vi "xy_ref_lpf.vi"(6 "enable":bool, 7 "lpf-Order":i32=2, 8 "Den":sgl[](array[numeric])=[0.982758, -1.98194, 1.0, 0.0, 0.0, 0.0, 0.0, 0.0, 0.0], 9 "Num":sgl[](array[numeric])=[-0.00254, 0.000408, 0.00295, 0.0, 0.0, 0.0, 0.0, 0.0, 0.0], 11 "xy_ref":fxp<+/-,16,5>[](array[numeric])=[0.0, 0.0]) -> (3 "xy_ref_filt":fxp<+/-,16,5>[](array[numeric]))   [LabVIEW 2017]
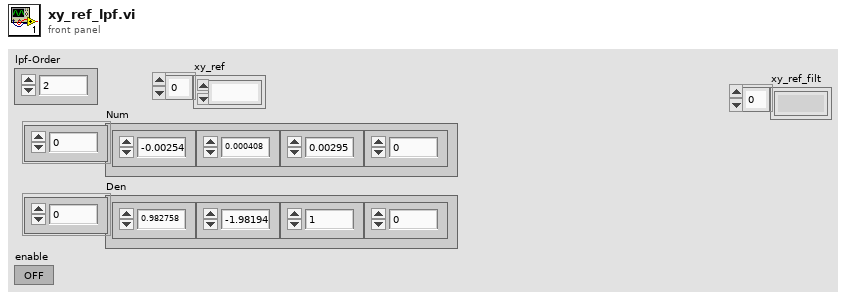
[diagram p1: front panel]
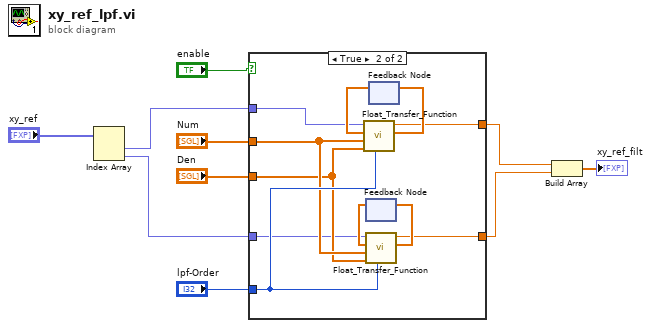
[diagram p0: block diagram]
diagram:
  n1 = Index Array(array="xy_ref") -> (element #1=w5:fxp<+/-,16,5>, element #2=w4:fxp<+/-,16,5>)  [unwired: 2 in]
  n2 = case shown="True" "enable" {
    tunnel: "lpf-Order" -> [_ w23]
    tunnel: "Num" -> [_ w22]
    tunnel: "Den" -> [_ w21]
    tunnel: [w12 w16] -> w2
    tunnel: [w11 w15] -> w1
    tunnel: w5 -> [w12 w14]
    tunnel: w4 -> [w11 w13]
    frame False {
    }
    frame True {
      n3 = feedback #1() -> (w19:sgl[])  [unwired: 1 in]
      n4 = call "Float_Transfer_Function.vi"("TF Order"=w23, "Den"=w21, "Num"=w22, "State In"=w19, "Input"=w13) -> ("State Out"=w20:sgl[], "Output"=w15:sgl)  [unwired: 4 in]
      n5 = feedback-in #1(w20) -> ()
      n6 = feedback #2() -> (w17:sgl[])  [unwired: 1 in]
      n7 = call "Float_Transfer_Function.vi"("TF Order"=w23, "Den"=w21, "Num"=w22, "State In"=w17, "Input"=w14) -> ("State Out"=w18:sgl[], "Output"=w16:sgl)  [unwired: 4 in]
      n8 = feedback-in #2(w18) -> ()
    }
  }
  n9 = Build Array(w2, w1) -> (→"xy_ref_filt":sgl[])
